vi "Calibrate Speed 2 Ticks (uSMC).vi"(1 "Index":i32, 2 "speed value (units)":dbl) -> (0 "speed ticks":u16)   [LabVIEW 2010, in "SignalWriterMH110203USBStepperMotor.lvclass"]
uses:
  SignalWriterMH110203USBStepperMotor.lvclass
  class_data.vi
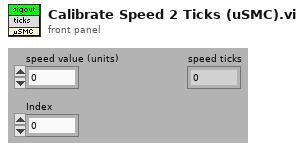
[diagram p1: front panel]
types:
  T1 = typedef "SignalWriterMH110203USBStepperMotor.lvclass/GoTo Control (uSMC).ctl" = cluster{"Step motor ID":string, "SMname":string, "Backlash":u16, "wait for input sygnal to start":bool, "use slow start/stop":bool, "units name":string, "Maximum speed":dbl, "speed":dbl, "step":u8, "point 1 ticks":i32, "point 2 ticks":i32, "point 1 units":dbl, "point 2 units":dbl, "Limit Switch standoff":dbl, "Zero Value":dbl, "Destination Position":dbl, "force backlash":bool, "power off when stop":bool, "POff delay":dbl, "positioner name":string, "R, Ohm":dbl, "I, mA":dbl, "Positioner's Type":u16, "Reset Direction":bool, "Manufacturer":string, "Model":string, "Scheme":string, "FirmwareVer":string}
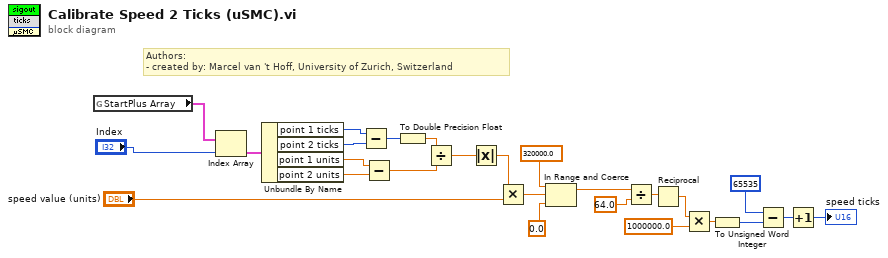
[diagram p0: block diagram]
diagram:
  # "Authors: \n- created by: Marcel van 't Hoff, University of Zurich, Switzerland"
  n1 = global read "class_data.vi" "StartPlus Array"() -> (w19:T1[])
  n2 = Index Array(array=w19, index="Index") -> (element=w18:T1)
  n3 = Unbundle By Name(w18) -> ("point 1 ticks"=w16:i32, "point 2 ticks"=w15:i32, "point 1 units"=w14:dbl, "point 2 units"=w13:dbl)
  n4 = Subtract(x=w16, y=w15) -> (x-y=w11:i32)
  n5 = Subtract(x=w14, y=w13) -> (x-y=w12:dbl)
  n6 = To Double Precision Float(number=w11) -> (double precision float=w10:dbl)
  n7 = Divide(x=w10, y=w12) -> (x/y=w9:dbl)
  n8 = Absolute Value(x=w9) -> (abs(x)=w2:dbl)
  n9 = Multiply(x=w2, y="speed value (units)") -> (x*y=w3:dbl)
  n10 = In Range and Coerce(upper limit=320000.0, x=w3, lower limit=0.0) -> (coerced(x)=w4:dbl)  [unwired: 1 out]
  n11 = Divide(x=w4, y=64.0 ("x")) -> (x/y=w7:dbl)
  n12 = Reciprocal(x=w7) -> (1/x=w24:dbl)
  n13 = Multiply(x=w24, y=1000000.0) -> (x*y=w20:dbl)
  n14 = To Unsigned Word Integer(number=w20) -> (unsigned 16bit integer=w22:u16)
  n15 = Subtract(x=u16 65535, y=w22) -> (x-y=w25:u16)
  n16 = Increment(x=w25) -> (x+1=→"speed ticks":u16)
